vi "ITestSettings No Configuration Error Generator.vi"(8 "error in (no error)":errorcluster, 10 "Configuration In":string, 11 "ITestSettings in":refnum<class "ITestSettings.lvclass">) -> (0 "error out":errorcluster, 3 "ITestSettings out":refnum<class "ITestSettings.lvclass">)   [LabVIEW 2016, in "ITestSettings.lvlib" / "ITestSettings.lvclass"]
uses:
  ITestSettings.lvclass
  ITestSettings.lvclass/ITestSettings.ctl
  Read Configuration Dictionary.vi
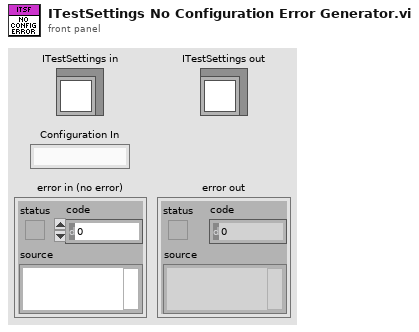
[diagram p1: front panel]
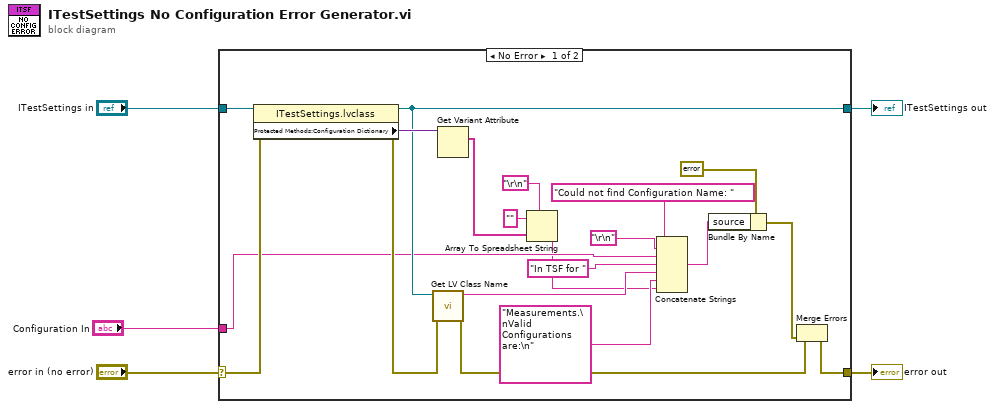
[diagram p0: block diagram]
diagram:
  n1 = case shown="No Error" "error in (no error)" {
    selector: "error in (no error)" -> [w16 w27]
    tunnel: [w6 w27] -> w4
    tunnel: [w17 w26] -> w2
    tunnel: "ITestSettings in" -> [w25 w26]
    tunnel: "Configuration In" -> [w14 _]
    frame No Error {
      n2 = property class="ITestSettings.lvclass"(reference=w25, error in=w16) -> (reference out=w17:refnum<class "ITestSettings.lvclass">, error out=w15:errorcluster, "Protected Methods:Configuration Dictionary"=w24:variant)
      n3 = call <vilib>:"Get LV Class Name.vi"("error in (no error)"=w15, "object"=w17) -> ("error out"=w8:errorcluster, "class name"=w11:string)  [unwired: 8 in]
      n4 = Get Variant Attribute(Variant=w24) -> (names=w23:string[])  [unwired: 3 in, 3 out]
      n5 = Array To Spreadsheet String(delimiter (Tab)="\r\n", array=w23, 3:"" ("format string")) -> (spreadsheet string=w9:string)
      n6 = Concatenate Strings("Could not find Configuration Name: ", "\r\n", w14, "In TSF for ", w11, "Measurements.\nValid Configurations are:\n", w9) -> (w19:string)
      n7 = Bundle By Name(cluster=errorcluster {"status"=TRUE, "code"=9002, "source"=""} ("error constant"), "source"=w19) -> (w7:errorcluster)
      n8 = Merge Errors(w8, w7) -> (w6:errorcluster)
    }
    frame Error {
    }
  }
  "error out" <- w4
  "ITestSettings out" <- w2
